vi "Logger Manual Entry.vi"(11 "error in (no error)":errorcluster) -> (15 "error out":errorcluster)   [LabVIEW 2018]
uses:
  Logger Global.vi
panel:
  in  "Log File Input":T1
  in  "EXIT":bool
  in  "Enter":bool
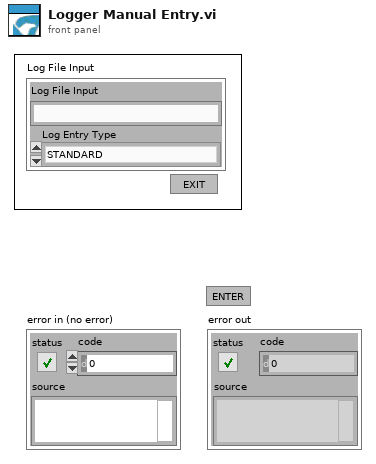
[diagram p1: front panel]
types:
  T1 = cluster{"Log File Input":string, "Log Entry Type":enum16{"STANDARD", "WARNING", "CRITICAL"}}
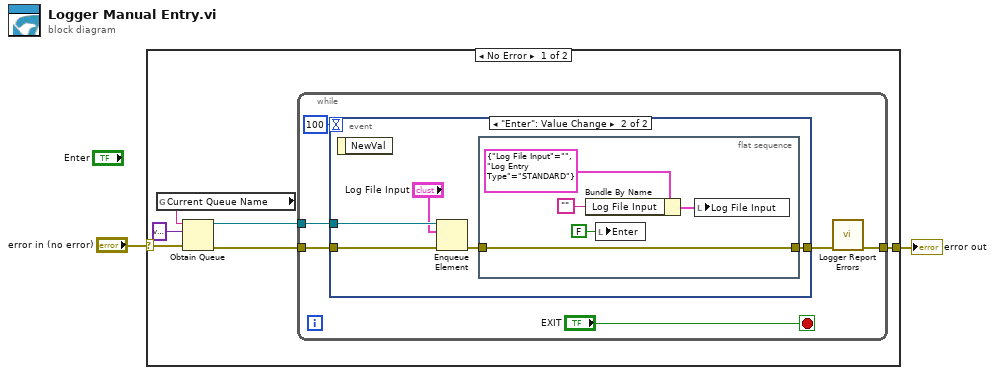
[diagram p0: block diagram]
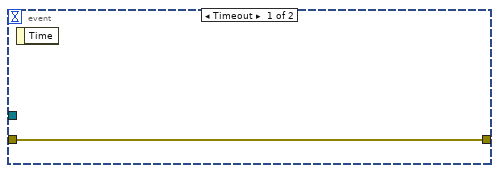
[diagram p2: hidden frame]
diagram:
  n1 = case shown="No Error" "error in (no error)" {
    selector: "error in (no error)" -> [w8 w26]
    tunnel: [w3 w26] -> w1
    frame No Error {
      n2 = global read "Logger Global.vi" "Current Queue Name"() -> (w5:string)
      n3 = Obtain Queue(name (unnamed)=w5, element data type=variant, error in (no error)=w8) -> (queue out=w6:refnum<queue>, error out=w7:errorcluster)  [unwired: 2 in, 1 out]
      n4 = while {
        tunnel: w6 -> [w13]
        tunnel: w7 -> [w14]
        tunnel: [w9] -> w3
        stop <- "EXIT" stop-if-true
        n5 = event shown="[1] \"Enter\": Value Change" {
          selector: _ -> [_ _]
          dyn-events: _ -> [_ _]
          timeout: 100 -> [_ _]
          tunnel: [w15 w17] -> w10
          tunnel: w14 -> [w15 w20]
          tunnel: w13 -> [_ w19]
          event Timeout {
            n6 = event-data() -> ()  [unwired: 1 in, 1 out]
          }
          event "Enter": Value Change {
            n7 = event-data() -> ()  [unwired: 1 in, 1 out]
            n8 = Enqueue Element(queue=w19, element="Log File Input", error in (no error)=w20) -> (error out=w18:errorcluster)  [unwired: 1 in, 2 out]
            n9 = flat-sequence {
              tunnel: [w25] -> w17
              tunnel: w18 -> [w25]
              frame #0 {
                n10 = Bundle By Name(cluster=T1 {"Log File Input"="", "Log Entry Type"=enum."STANDARD"} ("Log File Input"), "Log File Input"="") -> (w22:T1)
                n11 = local write "Enter"(FALSE ("Enter")) -> ()
                n12 = local write "Log File Input"(w22) -> ()
              }
            }
          }
        }
        n13 = call "Logger Report Errors.vi"("error in (no error)"=w10) -> ("error out"=w9:errorcluster)  [unwired: 14 in]
      }
    }
    frame Error {
    }
  }
  "error out" <- w1
